vi "NBFM Modulation Demo (Single Tone) - Music.vi"() -> ()   [LabVIEW 2013]
uses:
  <vilib>/sound2/lvsound2.llb/Sound File Info (path).vi
  <vilib>/sound2/lvsound2.llb/Sound File Read Open.vi
  <vilib>/sound2/lvsound2.llb/Sound File Read (DBL).vi
  <vilib>/Waveform/WDTOps.llb/WDT Get Waveform Subset DBL.vi
  <vilib>/addons/Modulation/Analog/MT Passband PLL.vi
  <vilib>/express/express analysis/Spectral/Block/exnSpectralBlock spectral measurements power poly.vi
  <vilib>/express/express analysis/Spectral/Block/exnSpectralBlock spectral measurements power DDT.vi
  <vilib>/express/express analysis/Spectral/XNode/ExpressSpectralMeasurementsBlockNode.xnode
  <vilib>/addons/Modulation/niAMT.lvlib
  <vilib>/Analysis/NI_AALPro.lvlib
panel:
  in  "Path":path=path "D:/wendy/study/2023-2024Spring/EE206lab/lab4/mozart.wav"
  in  "Duration":dbl=44101.0 caption="Frequency"
  in  "Resample Rate":dbl=1000000.0 caption="Frequency"
  out "estimated carrier frequency (Hz)":dbl
  in  "WAV SR":dbl=44100.0 caption="dt"
  in  "LPF Cut-Off":dbl=10000.0 caption="Lower Cut-Off"
  in  "AWGN (dB)":dbl(slide)=30.0 caption="Standard deviation" scale=-20.0..50.0
  out "Recovered Signal":dynamicdata(graph)
  out "Baseband":dynamicdata(graph)
  out "FM FFT":dynamicdata(graph)
  out "FM Wave":dynamicdata(graph)
  in  "Carrier Amp.":dbl=1.0 caption="Amplitude"
  in  "stop":bool
  in  "Frequency Deviation":dbl(slide)=400.0 scale=0.0..400.0
  in  "Carrier Freq.":dbl=100000.0 caption="Frequency"
  # "Frequency Modulation"
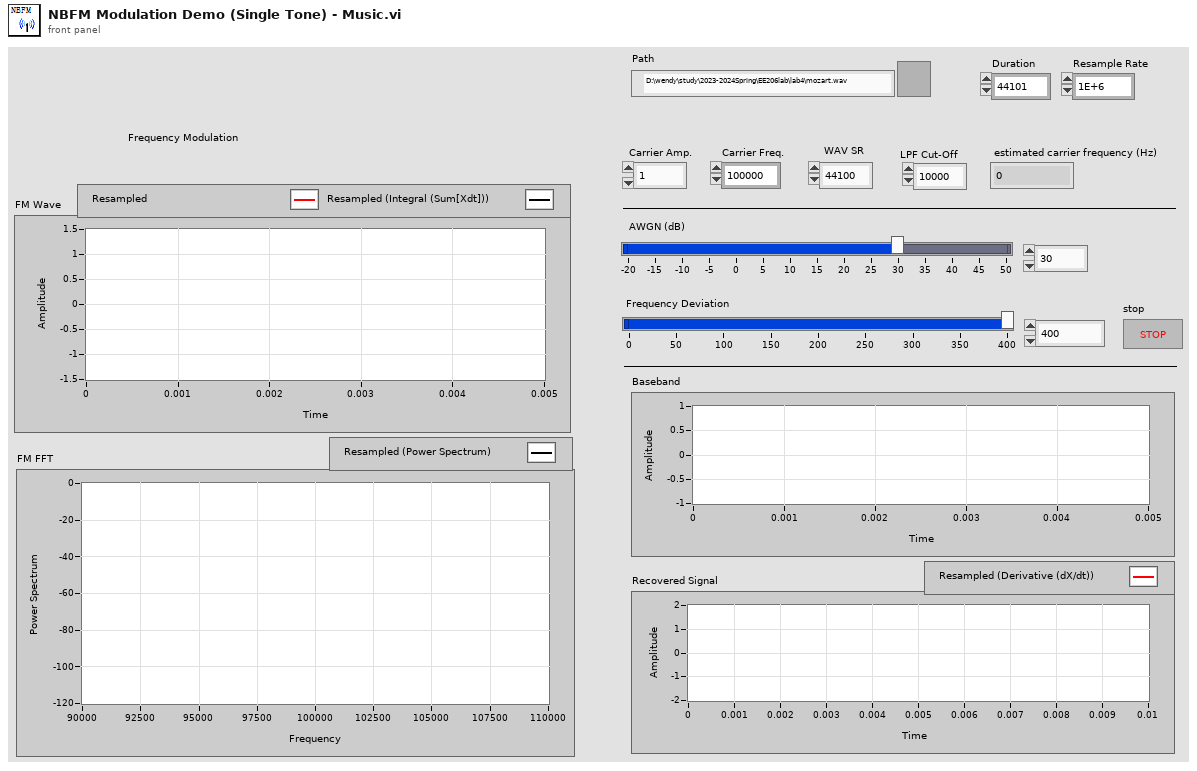
[diagram p1: front panel]
types:
  T1 = typedef "Sound File Refnum.ctl" = refnum<file>
  T2 = cluster{"averaging mode":u16, "weighting mode":u16, "number of averages":u32}
  T3 = cluster{"dB On (F)":bool, "unwrap phase (F)":bool, "convert to degree (F)":bool}
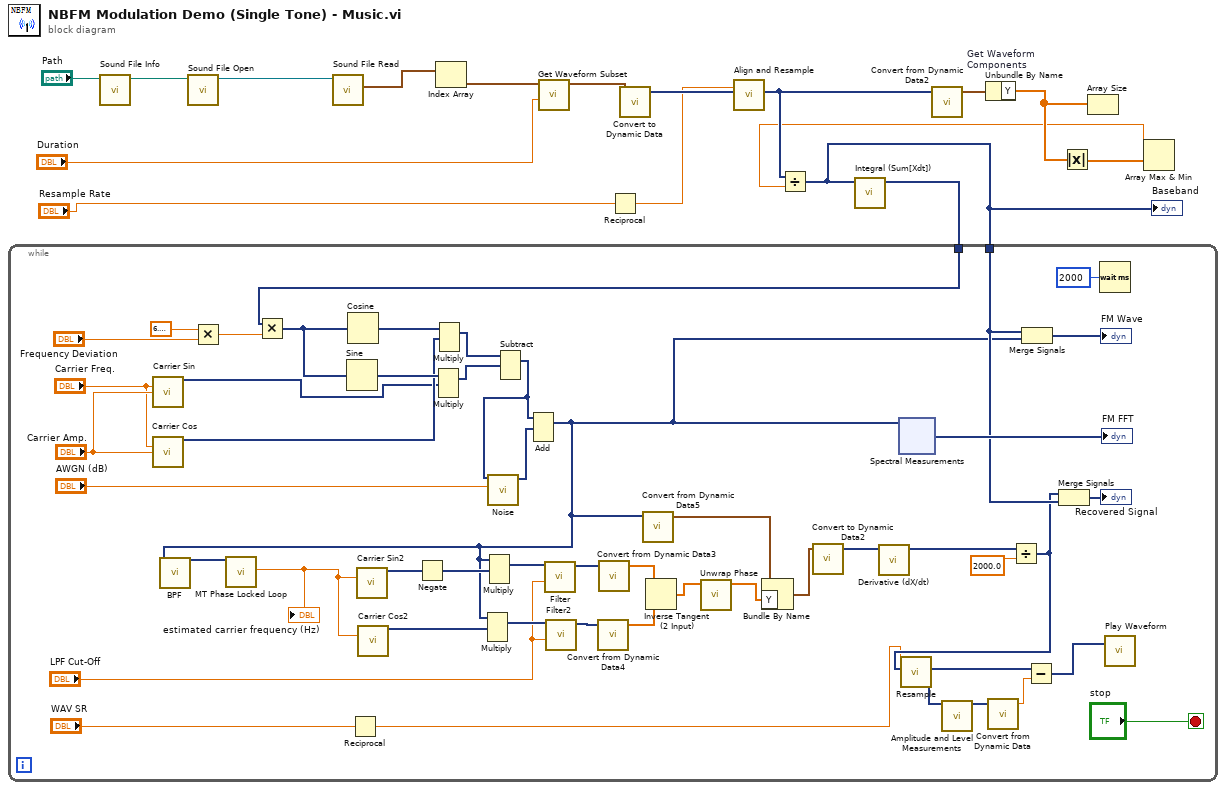
[diagram p0: block diagram]
diagram:
  n1 = call-poly <vilib>:"Sound File Info.vi"("path"="Path") -> ("path out"=w8:path)  [unwired: 7 in, 3 out]
  n2 = call-poly <vilib>:"Sound File Open.vi"("path"=w8) -> ("sound file refnum"=w16:T1)  [unwired: 9 in, 1 out]
  n3 = call-poly <vilib>:"Sound File Read.vi"("sound file refnum"=w16) -> ("data"=w15:waveform(dbl)[])  [unwired: 6 in, 4 out]
  n4 = Index Array "Index Array"(array=w15) -> (element=w14:waveform(dbl))  [unwired: 1 in]
  n5 = call-poly <vilib>:"Get Waveform Subset.vi"("duration"="Duration", "waveform in"=w14) -> ("waveform out"=w9:waveform(dbl))  [unwired: 4 in, 3 out]
  n6 = Reciprocal(x="Resample Rate") -> (1/x=w10:dbl)
  n7 = call "Convert to Dynamic Data"("Waveform"=w9) -> ("Dynamic Data Type"=w13:dynamicdata)  [unwired: 3 in]
  n8 = call "Align and Resample"("dt"=w10, "Signals"=w13) -> ("Resampled Signals"=w4:dynamicdata)  [unwired: 7 in, 2 out]
  n9 = call "Convert from Dynamic Data2"("Dynamic Data Type"=w4) -> ("Waveform"=w7:waveform(dbl))  [unwired: 3 in]
  n10 = Unbundle By Name "Get Waveform Components"(w7) -> ("Y"=w12:dbl[])
  n11 = Absolute Value(x=w12) -> (abs(x)=w11:dbl[])
  n12 = Array Size(array=w12) -> ()  [unwired: 1 out]
  n13 = Array Max & Min(array=w11) -> (max value=w3:dbl)  [unwired: 3 out]
  n14 = Divide(x=w4, y=w3) -> (x/y=w1:dynamicdata)
  "Baseband" <- w1
  n15 = call "Integral (Sum[Xdt])"("Signals"=w1) -> ("Result"=w2:dynamicdata)  [unwired: 5 in, 1 out]
  n16 = while {
    tunnel: w1 -> [w35]
    tunnel: w2 -> [w49]
    stop <- "stop" stop-if-true
    n17 = call "Carrier Sin"("Frequency"="Carrier Freq.", "Amplitude"="Carrier Amp.") -> ("Sine"=w44:dynamicdata)  [unwired: 12 in, 1 out]
    n18 = call "Carrier Cos"("Frequency"="Carrier Freq.", "Amplitude"="Carrier Amp.") -> ("Sine"=w45:dynamicdata)  [unwired: 12 in, 1 out]
    n19 = Multiply(x=6.283185307179586, y="Frequency Deviation") -> (x*y=w61:dbl)
    n20 = Multiply(x=w49, y=w61) -> (x*y=w47:dynamicdata)
    n21 = Sine(x=w47) -> (sin(x)=w46:dynamicdata)
    n22 = Cosine(x=w47) -> (cos(x)=w48:dynamicdata)
    n23 = Reciprocal(x="WAV SR") -> (1/x=w32:dbl)
    n24 = Multiply(1:w44, 2:w46) -> (0:w42:dynamicdata)  [unwired: 1 in, 1 out]
    n25 = Multiply(1:w45, 2:w48) -> (0:w43:dynamicdata)  [unwired: 1 in, 1 out]
    n26 = Subtract(1:w42, 2:w43) -> (0:w40:dynamicdata)  [unwired: 1 in, 1 out]
    n27 = call "Noise.vi"("AWGN (dB)"="AWGN (dB)", "Dynamic Data"=w40) -> ("DC with Gaussian Noise"=w41:dynamicdata)  [unwired: 9 in]
    n28 = Add(1:w41, 2:w40) -> (0:w24:dynamicdata)  [unwired: 1 in, 1 out]
    n29 = call "BPF"("Signal"=w24) -> ("Filtered Signal"=w56:dynamicdata)  [unwired: 9 in, 1 out]
    n30 = call-poly <vilib>:"MT Phase Locked Loop.vi"("passband waveform"=w56) -> ("estimated carrier frequency (Hz)"=w39:dbl)  [unwired: 10 in, 4 out]
    "estimated carrier frequency (Hz)" <- w39
    n31 = call "Carrier Sin2"("Frequency"=w39) -> ("Sine"=w55:dynamicdata)  [unwired: 13 in, 1 out]
    n32 = call "Carrier Cos2"("Frequency"=w39) -> ("Sine"=w37:dynamicdata)  [unwired: 13 in, 1 out]
    n33 = Negate(x=w55) -> (-x=w38:dynamicdata)
    n34 = Multiply(1:w37, 2:w24) -> (0:w31:dynamicdata)  [unwired: 1 in, 1 out]
    n35 = Multiply(1:w38, 2:w24) -> (0:w30:dynamicdata)  [unwired: 1 in, 1 out]
    n36 = call "Filter"("Lower Cut-Off"="LPF Cut-Off", "Signal"=w30) -> ("Filtered Signal"=w28:dynamicdata)  [unwired: 8 in, 1 out]
    n37 = call "Filter2"("Lower Cut-Off"="LPF Cut-Off", "Signal"=w31) -> ("Filtered Signal"=w27:dynamicdata)  [unwired: 8 in, 1 out]
    n38 = call "Convert from Dynamic Data4"("Dynamic Data Type"=w27) -> ("Array"=w25:dbl[])  [unwired: 3 in]
    n39 = call "Convert from Dynamic Data3"("Dynamic Data Type"=w28) -> ("Array"=w26:dbl[])  [unwired: 3 in]
    n40 = call "Convert from Dynamic Data5"("Dynamic Data Type"=w24) -> ("Waveform"=w20:waveform(dbl))  [unwired: 3 in]
    n41 = Inverse Tangent (2 Input)(1:w25, 2:w26) -> (0:w22:dbl[])
    n42 = call <vilib>:"Unwrap Phase.vi"("Phase"=w22) -> ("Unwrapped Phase"=w21:dbl[])  [unwired: 9 in, 1 out]
    n43 = Bundle By Name(cluster=w20, "Y"=w21) -> (w19:waveform(dbl))
    n44 = call "Convert to Dynamic Data2"("Waveform"=w19) -> ("Dynamic Data Type"=w23:dynamicdata)  [unwired: 3 in]
    n45 = call "Derivative (dX/dt)"("Signals"=w23) -> ("Result"=w34:dynamicdata)  [unwired: 5 in, 1 out]
    n46 = xnode "Spectral Measurements"("Signals"=w24) -> ("Power Spectrum"=→"FM FFT":dynamicdata)  [unwired: 1 in, 1 out]
    n47 = Divide(x=w34, y=2000.0) -> (x/y=w33:dynamicdata)
    n48 = call "Resample"("dt"=w32, "Signals"=w33) -> ("Resampled Signals"=w52:dynamicdata)  [unwired: 7 in, 2 out]
    n49 = call "Amplitude and Level Measurements"("Signals"=w52) -> ("Mean (DC)"=w53:dynamicdata)  [unwired: 13 in, 1 out]
    n50 = call "Convert from Dynamic Data"("Dynamic Data Type"=w53) -> ("Scalar"=w51:dbl)  [unwired: 3 in]
    n51 = Merge Signals(w35, w24) -> (→"FM Wave":dynamicdata)
    n52 = Subtract(x=w52, y=w51) -> (x-y=w50:dynamicdata)
    n53 = Merge Signals(w33, w35) -> (→"Recovered Signal":dynamicdata)
    n54 = Wait (ms)(milliseconds to wait=u32 2000) -> ()  [unwired: 1 out]
    n55 = call "Play Waveform"("Data"=w50) -> ()  [unwired: 18 in, 1 out]
  }
